vi "Stop.vi"(8 "error in (no error)":errorcluster, 10 "Message in":refnum<class "StopMessage.lvclass">, 11 "Test_ExampleClassA in":refnum<class "Test_ExampleClassA.lvclass">) -> (0 "error out":errorcluster, 3 "Test_ExampleClassA out":refnum<class "Test_ExampleClassA.lvclass">)   [LabVIEW 2012, in "Test_ExampleClassA.lvclass"]
doc: "Called when the data streaming from the test subject has stopped."
uses:
  Test_ExampleClassA.lvclass
  StopMessage/StopMessage.lvclass
  MurmexTest/MurmexTest.lvclass
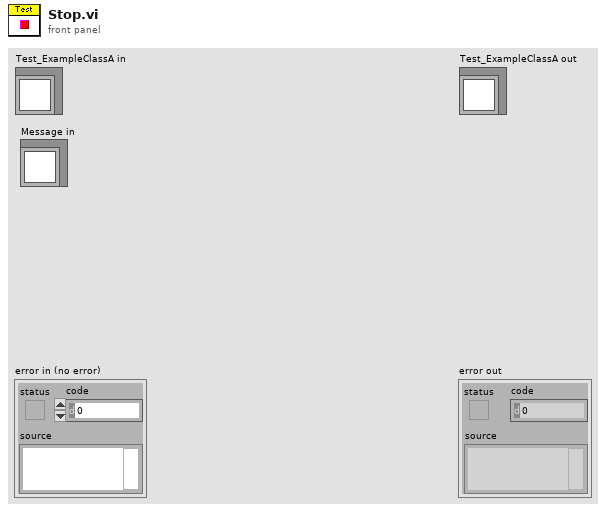
[diagram p1: front panel]
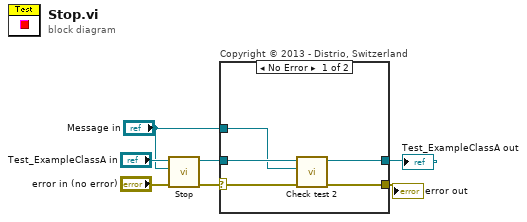
[diagram p0: block diagram]
diagram:
  n1 = call-parent "Stop.vi"("error in (no error)"="error in (no error)", "Message in"="Message in", "Murmex in"="Test_ExampleClassA in") -> ("error out"=w5:errorcluster, "Murmex out"=w4:refnum<class "Test_ExampleClassA.lvclass">)  [unwired: 7 in]
  n2 = case "Copyright © 2013 - Distrio, Switzerland" shown="No Error" w5 {
    selector: w5 -> [w11 w13]
    tunnel: w4 -> [w12 w14]
    tunnel: "Message in" -> [w10 _]
    tunnel: [w9 w14] -> w2
    tunnel: [w8 w13] -> w1
    frame No Error {
      n3 = call "Check test 2.vi"("error in (no error)"=w11, "Message in"=w10, "Test_ExampleClassA in"=w12) -> ("error out"=w8:errorcluster, "Test_ExampleClassA out"=w9:refnum<class "Test_ExampleClassA.lvclass">)  [unwired: 7 in]
    }
    frame Error {
    }
  }
  "error out" <- w1
  "Test_ExampleClassA out" <- w2
